vi "TSM SSC Digital Fetch Capture Waveform.vi"(0 "Digital TSM In":T1, 1 "Waveform Name":string, 7 "timeout (s)":dbl=10.0, 9 "samples to read":i32, 11 "error in":errorcluster) -> (4 "Digital TSM Out":T1, 6 "Per-Site Waveforms":u32[][](array[numeric]) format="%.0x", 15 "error out":errorcluster)   [LabVIEW 2020]
doc: "Fetches a defined number of samples for the sites connected to the specified pin(s) and pin group(s). This VI only returns data from sites that are enabled when fetch is called. Returns an array of per-site per-sample data where rows correspond to sites and columns correspond to samples."
uses:
  TSM/TSM SSC Digital.ctl
  <vilib>/NI_TestStand_SemiconductorModule/NI_TestStand_Semiconductor_Module.lvlibp/PinMap/Digital Pattern/PinQueryContext/DigitalPatternPinQueryContext.lvclass
  SSC Digital/SSC Digital.ctl
  0d73af61-f07e-44ac-906d-5bf207f8a2bd.vi
  Shared SubVIs/Site List to Site Numbers.vi
  Shared SubVIs/Trim Whitespace [Inlined].vi
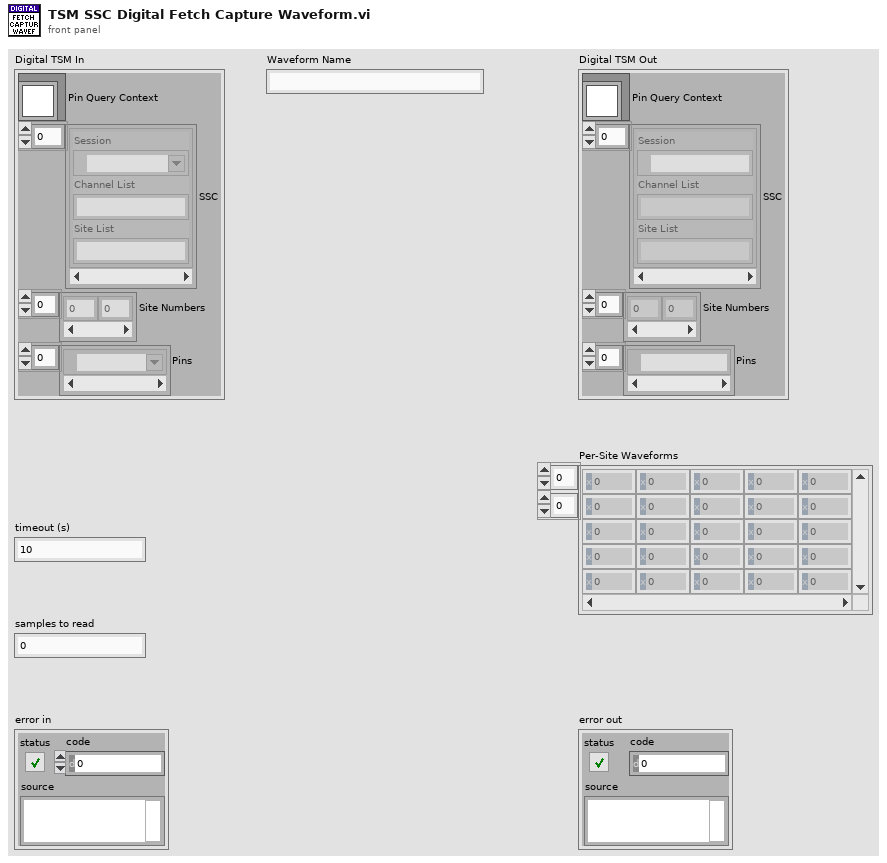
[diagram p1: front panel]
types:
  T1 = typedef "TSM SSC Digital.ctl" = cluster{"Pin Query Context":refnum<class "DigitalPatternPinQueryContext.lvclass">, "SSC":T2[], "Site Numbers":i32[], "Pins":tag[]}
  T2 = typedef "SSC Digital.ctl" = cluster{"Session":refnum<k15>, "Channel List":string, "Site List":string}
  T3 = typedef "Digital 1D Location Array in a Cluster.ctl" = cluster{"Digital 1D Location Array":i32[]}
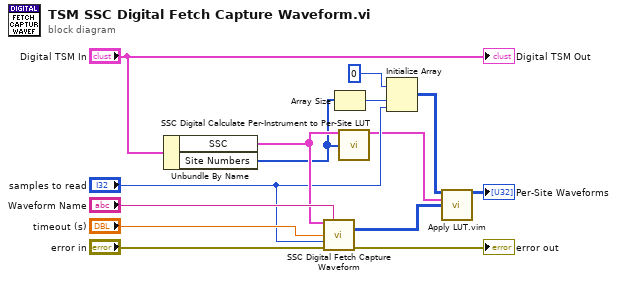
[diagram p0: block diagram]
diagram:
  n1 = Unbundle By Name("Digital TSM In") -> ("SSC"=w10:T2[], "Site Numbers"=w1:i32[])
  n2 = call "SSC Digital Fetch Capture Waveform.vi"("Digital SSC in"=w10, "Waveform Name"="Waveform Name", "timeout (s)"="timeout (s)", "samples to read"="samples to read", "error in"="error in") -> ("Per-Instrument Capture"=w5:u32[][][], "error out"=→"error out":errorcluster)  [unwired: 8 in, 1 out]
  n3 = Array Size(array=w1) -> (size(s)=w9:i32)
  n4 = call "SSC Digital Calculate Per-Instrument to Per-Site LUT.vi"("Digital SSC In"=w10, "Sites"=w1) -> ("Per-Instrument to Per-Site LUT"=w4:T3[])  [unwired: 13 in]
  n5 = Initialize Array(u32 0, w9, "samples to read") -> (w6:u32[][])
  n6 = call "Apply LUT.vim"("Initialized Array"=w6, "LUT"=w4, "Results to Apply LUT to"=w5) -> ("Array Out"=→"Per-Site Waveforms":u32[][])  [unwired: 12 in]
  "Digital TSM Out" <- "Digital TSM In"
